vi "LoggingMain.vi"(8 "Operation":T1, 10 "Data":variant, 11 "Name":string) -> (3 "Log String":string)   [LabVIEW 2017]
uses:
  LogOperation.ctl
  <vilib>/Utility/Data Type/NI_Data Type.lvlib
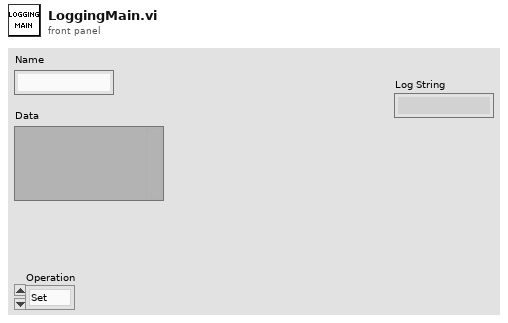
[diagram p1: front panel]
types:
  T1 = typedef "LogOperation.ctl" = enum16{"Set", "Get All", "Init"}
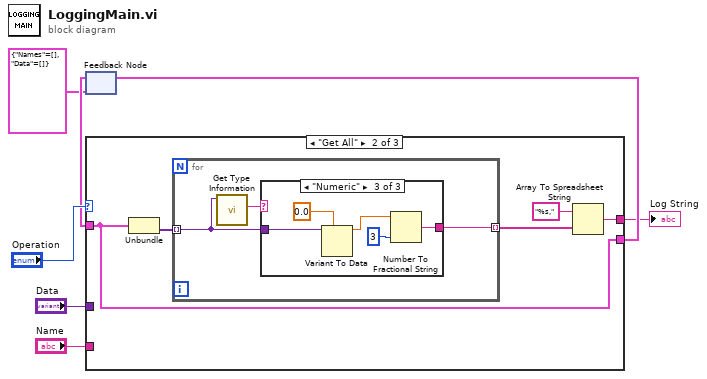
[diagram p0: block diagram]
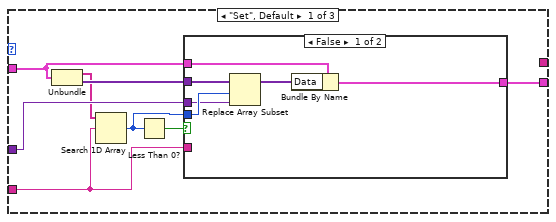
[diagram p2: hidden frame]
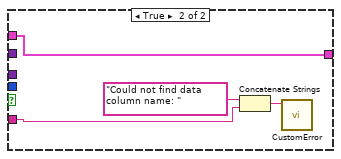
[diagram p3: hidden frame]
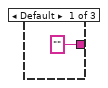
[diagram p4: hidden frame]
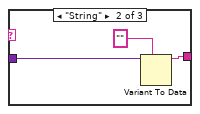
[diagram p5: hidden frame]
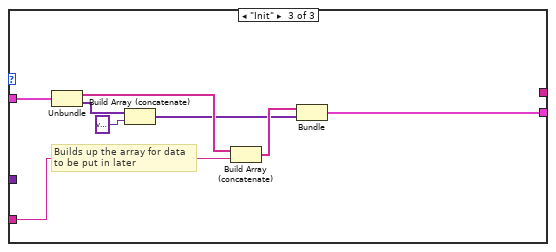
[diagram p6: hidden frame]
diagram:
  n1 = feedback #1(cluster{"Names":string[], "Data":variant[]} {"Names"=[], "Data"=[]}) -> (w6:cluster{"Names":string[], "Data":variant[]})
  n2 = case shown="\"Get All\"" "Operation" {
    tunnel: w6 -> [w8 w30 w50]
    tunnel: [w9 w30 w43] -> w3
    tunnel: "Name" -> [w14 _ w46]
    tunnel: "Data" -> [w11 _ _]
    tunnel: [_ w27 _] -> w1
    frame "Set", Default {
      n3 = Unbundle(w8) -> ("Names"=w10:string[], "Data"=w13:variant[])
      n4 = Search 1D Array(1D array=w10, element=w14) -> (index of element=w12:i32)  [unwired: 1 in]
      n5 = Less Than 0?(x=w12) -> (x < 0?=w15:bool)
      n6 = case shown="False" w15 {
        tunnel: w14 -> [_ w23]
        tunnel: w13 -> [w21 _]
        tunnel: w12 -> [w20 _]
        tunnel: w11 -> [w19 _]
        tunnel: [w16 w22] -> w9
        tunnel: w8 -> [w18 w22]
        frame False {
          n7 = Replace Array Subset(array=w21, new element=w19, index=w20) -> (w17:variant[])
          n8 = Bundle By Name(cluster=w18, "Data"=w17) -> (w16:cluster{"Names":string[], "Data":variant[]})
        }
        frame True {
          n9 = Concatenate Strings("Could not find data column name: ", w23) -> (w24:string)
          n10 = call "CustomError.vi"("String"=w24) -> ()  [unwired: 10 in, 1 out]
        }
      }
    }
    frame "Get All" {
      n11 = Unbundle(w30) -> ("Data"=w29:variant[])  [unwired: 1 out]
      n12 = for {
        tunnel: w29 -> [w31] mode=indexing
        tunnel: [w32] -> w26 mode=indexing
        n13 = call <vilib>:"Get Type Information.vi"("Variant"=w31) -> ("Name"=w33:string)  [unwired: 6 in, 4 out]
        n14 = case shown="\"Numeric\"" w33 {
          tunnel: ["" ("Name") w36 w38] -> w32
          tunnel: w31 -> [_ w37 w42]
          frame Default {
          }
          frame "String" {
            n15 = Variant To Data(type="" ("Name"), Variant=w37) -> (data=w36:string)  [unwired: 1 in, 1 out]
          }
          frame "Numeric" {
            n16 = Variant To Data(type=0.0, Variant=w42) -> (data=w40:dbl)  [unwired: 1 in, 1 out]
            n17 = Number To Fractional String(number=w40, precision (6)=i16 3) -> (F-format string=w38:string)  [unwired: 2 in]
          }
        }
      }
      n18 = Array To Spreadsheet String(array=w26, 3:"%s," ("format string")) -> (spreadsheet string=w27:string)  [unwired: 1 in]
    }
    frame "Init" {
      # "Builds up the array for data\nto be put in later"
      n19 = Unbundle(w50) -> ("Names"=w49:string[], "Data"=w48:variant[])
      n20 = Build Array (concatenate)(w48, variant ("Data")) -> (w44:variant[])
      n21 = Build Array (concatenate)(w49, w46) -> (w45:string[])
      n22 = Bundle(w45, w44) -> (w43:cluster{string[], variant[]})  [unwired: 1 in]
    }
  }
  "Log String" <- w1
  n23 = feedback-in #1(w3) -> ()
